vi "DAQDigital_Examples.vi"() -> ()   [LabVIEW 2020]
uses:
  <vilib>/DAQmx/read.llb/DAQmx Read (Digital 1D Bool NChan 1Samp 1Line).vi
  <vilib>/DAQmx/read.llb/DAQmx Read (Digital 1D U32 NChan 1Samp).vi
  <vilib>/DAQmx/miscellaneous.llb/DAQmx Fill In Error Info.vi
panel:
  out "Boolean array":bool[](array[boolean])
  out "Waveform Chart":u32[](graph)
  out "error out":errorcluster
  in  "DAQ Board Name Ports":tag
  in  "Channels Ports":tag[](array[tag])
  in  "error in":errorcluster
  in  "stop ports acquisition":bool
  out "error out 2":errorcluster
  in  "error in 2":errorcluster caption="error in"
  in  "Channels Lines":tag[](array[tag])
  in  "DAQ Board Name 2":tag
  in  "stop lines acquisition":bool
  out "data":bool[](array[boolean])
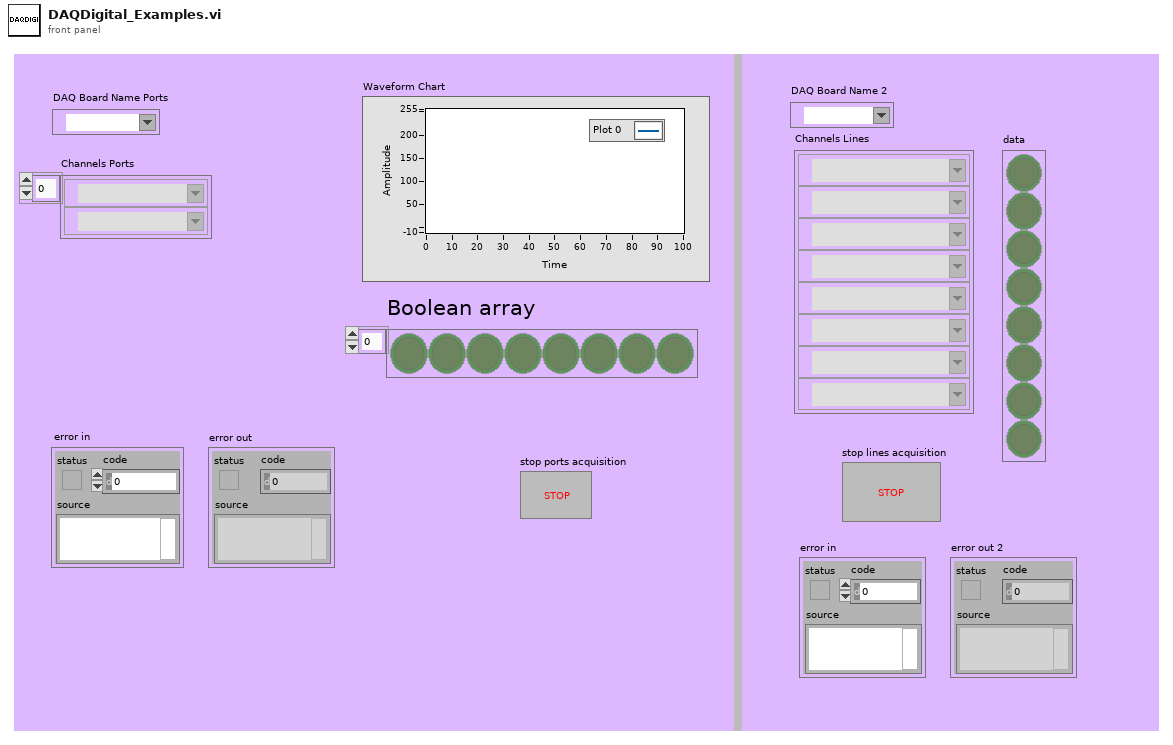
[diagram p1: front panel]
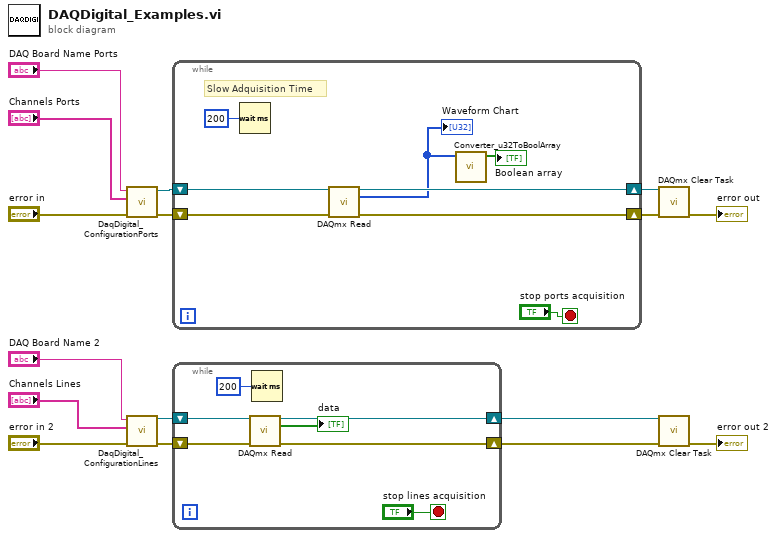
[diagram p0: block diagram]
diagram:
  n1 = call "DaqDigital_ConfigurationPorts.vi"("error in"="error in", "Canales"="Channels Ports", "DAQ Board Name"="DAQ Board Name Ports") -> ("error out"=w10:errorcluster, "task out"=w11:refnum<k21>)  [unwired: 7 in]
  n2 = call "DaqDigital_ConfigurationLines.vi"("error in"="error in 2", "Canales"="Channels Lines", "DAQ Board Name"="DAQ Board Name 2") -> ("error out"=w6:errorcluster, "task out"=w7:refnum<k21>)  [unwired: 7 in]
  n3 = while {
    shift-right: [w20] -> w13
    shift-left: w11 -> [w23]
    shift-right: [w19] -> w12
    shift-left: w10 -> [w22]
    stop <- "stop ports acquisition" stop-if-true
    # "Slow Adquisition Time"
    n4 = Wait (ms)(milliseconds to wait=u32 200) -> ()  [unwired: 1 out]
    n5 = call-poly <vilib>:"DAQmx Read.vi"("task/channels in"=w23, "error in"=w22) -> ("task out"=w20:refnum<k21>, "data"=w18:u32[], "error out"=w19:errorcluster)  [unwired: 11 in]
    "Waveform Chart" <- w18
    n6 = call "Converter_u32ToBoolArray.vi"("data"=w18) -> ("Boolean array"=→"Boolean array":bool[])  [unwired: 10 in]
  }
  n7 = while {
    shift-right: [w30] -> w8
    shift-left: w7 -> [w29]
    shift-right: [w31] -> w9
    shift-left: w6 -> [w28]
    stop <- "stop lines acquisition" stop-if-true
    n8 = call-poly <vilib>:"DAQmx Read.vi"("task/channels in"=w29, "error in"=w28) -> ("task out"=w30:refnum<k21>, "data"=→"data":bool[], "error out"=w31:errorcluster)  [unwired: 11 in]
    n9 = Wait (ms)(milliseconds to wait=u32 200) -> ()  [unwired: 1 out]
  }
  n10 = call <vilib>:"DAQmx Clear Task.vi"("task in"=w13, "error in"=w12) -> ("error out"=→"error out":errorcluster)  [unwired: 13 in]
  n11 = call <vilib>:"DAQmx Clear Task.vi"("task in"=w8, "error in"=w9) -> ("error out"=→"error out 2":errorcluster)  [unwired: 13 in]
